vi "Write CompressorDevRef.vi"(8 "error in (no error)":errorcluster, 10 "CompressorDevRef":T1={"DevStatus"={"status"=FALSE, "code"=0, "source"=""}, "DigitalInputDevRef"={"DevStatus"={"status"=FALSE, "code"=0, "source"=""}, "DIO Channel"=enum."DIO 3", "Digital Module"=enum."Digital Module 1"}, "RelayDevRef"={"DevStatus"={"status"=FALSE, "code"=0, "source"=""}, "Relay Channel"=enum."Relay 2", "Digital Module"=enum."Digital Module 1", "Relay Direction"=enum."Both directions"}}, 11 "Compressor in":refnum<class "Compressor.lvclass">) -> (0 "error out":errorcluster, 3 "Compressor out":refnum<class "Compressor.lvclass">)   [LabVIEW 2013, in "Compressor.lvclass"]
uses:
  Compressor.lvclass
  <vilib>/Rock Robotics/WPI/Compressor/WPI_CompressorDevRef.ctl
  <vilib>/Rock Robotics/WPI/DigitalInput/WPI_DigitalInputDevRef.ctl
  <vilib>/Rock Robotics/SystemInterfaces/DIO/FPGA_DIOChannel.ctl
  <vilib>/Rock Robotics/SystemInterfaces/Typedef/FPGA_TypedefDigitalModule.ctl
  <vilib>/Rock Robotics/WPI/Relay/WPI_RelayDevRef.ctl
  <vilib>/Rock Robotics/SystemInterfaces/DIO/FPGA_DIORelayChannel.ctl
  <vilib>/Rock Robotics/WPI/Relay/WPI_RelayDirection.ctl
  Compressor.lvclass/Compressor.ctl
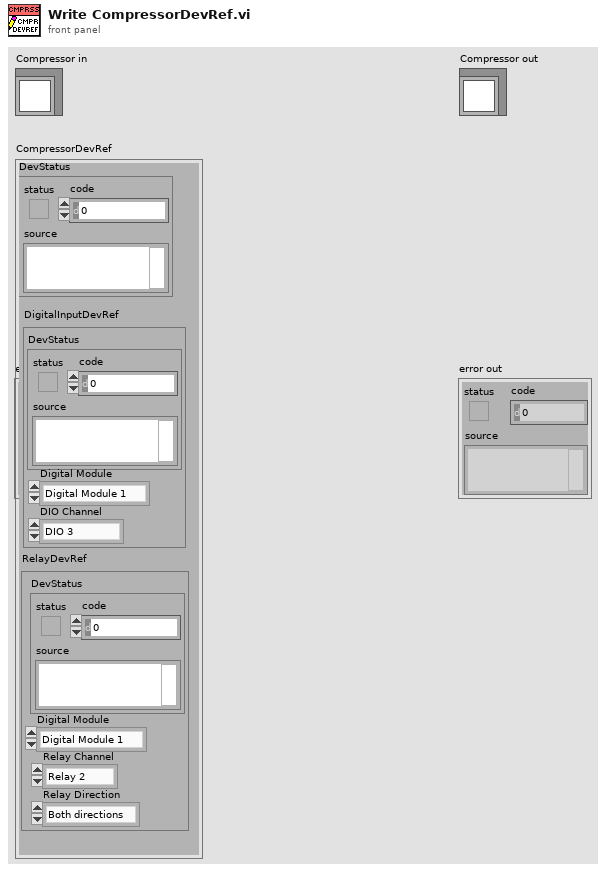
[diagram p1: front panel]
types:
  T1 = typedef "WPI_CompressorDevRef.ctl" = cluster{"DevStatus":errorcluster, "DigitalInputDevRef":T2, "RelayDevRef":T5}
  T2 = typedef "WPI_DigitalInputDevRef.ctl" = cluster{"DevStatus":errorcluster, "DIO Channel":T3, "Digital Module":T4}
  T3 = typedef "FPGA_DIOChannel.ctl" = enum8{"DIO 1", "DIO 2", "DIO 3", "DIO 4", "DIO 5", "DIO 6", "DIO 7", "DIO 8", "DIO 9", "DIO 10", "DIO 11", "DIO 12", "DIO 13", "DIO 14", "Invalid"}
  T4 = typedef "FPGA_TypedefDigitalModule.ctl" = enum16{"Digital Module 1", "Digital Module 2"}
  T5 = typedef "WPI_RelayDevRef.ctl" = cluster{"DevStatus":errorcluster, "Relay Channel":T6, "Digital Module":T4, "Relay Direction":T7}
  T6 = typedef "FPGA_DIORelayChannel.ctl" = enum8{"Relay 1", "Relay 2", "Relay 3", "Relay 4", "Relay 5", "Relay 6", "Relay 7", "Relay 8", "Invalid"}
  T7 = typedef "WPI_RelayDirection.ctl" = enum16{"Both directions", "Forward only", "Reverse only"}
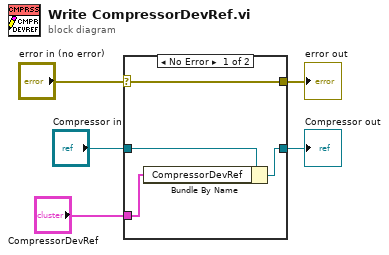
[diagram p0: block diagram]
diagram:
  n1 = case shown="No Error" "error in (no error)" {
    selector: "error in (no error)" -> [w9 w10]
    tunnel: [w9 w10] -> w4
    tunnel: [w7 w11] -> w2
    tunnel: "Compressor in" -> [w8 w11]
    tunnel: "CompressorDevRef" -> [w6 _]
    frame No Error {
      n2 = Bundle By Name(cluster=w8, "CompressorDevRef"=w6) -> (w7:refnum<class "Compressor.lvclass">)
    }
    frame Error {
    }
  }
  "error out" <- w4
  "Compressor out" <- w2
